vi "iStep.CreateSetpoints.vi"(11 "Parameters":dbl[](array[numeric])) -> (2 "samples":i32, 3 "iStep Pattern":dbl[](array[numeric]))   [LabVIEW 2015, in "Single Station Execution.lvlib"]
uses:
  Single Station Execution.lvlib
  <vilib>/Analysis/1siggen.llb/Ramp Pattern by Delta.vi
  <vilib>/Analysis/NI_AALBase.lvlib
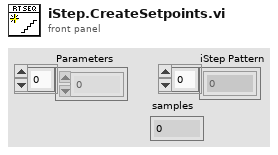
[diagram p1: front panel]
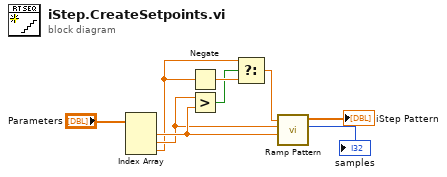
[diagram p0: block diagram]
diagram:
  n1 = Index Array(array="Parameters") -> (element #1=w9:dbl, element #2=w8:dbl, element #3=w6:dbl)  [unwired: 3 in]
  n2 = Negate(x=w6) -> (-x=w5:dbl)
  n3 = Greater?(x=w8, y=w9) -> (0:w4:bool)
  n4 = Select(t=w6, s=w4, f=w5) -> (s? t:f=w7:dbl)
  n5 = call-poly <vilib>:"Ramp Pattern.vi"("start"=w9, "end"=w8, "delta"=w7) -> ("samples"=→"samples":i32, "Ramp Pattern"=→"iStep Pattern":dbl[])  [unwired: 6 in, 1 out]
